vi "Position Arming LED.vi"(8 "error in (no error)":errorcluster, 9 "GPS Status LED":refnum<vi>, 10 "Aircraft Id Ref":refnum<vi>, 11 "LED Ref":refnum<vi>) -> (0 "error out":errorcluster)   [LabVIEW 2014]
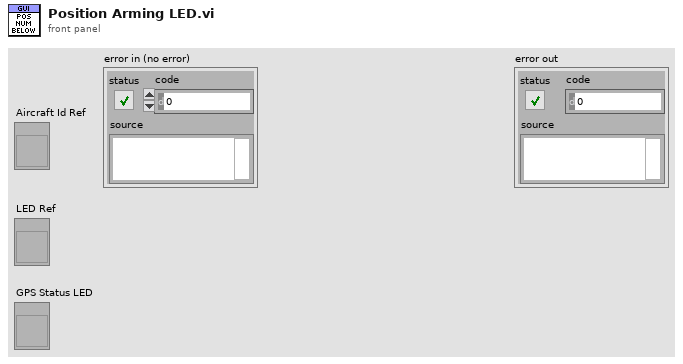
[diagram p1: front panel]
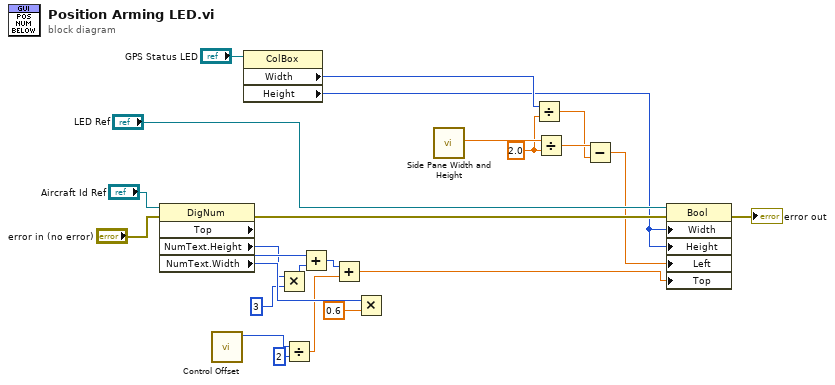
[diagram p0: block diagram]
diagram:
  w4 = 2.0 ("y")
  n1 = property class="DigNum"(reference="Aircraft Id Ref", error in="error in (no error)") -> (error out=w24:errorcluster, "Top"=w23:i32, "NumText.Height"=w14:u32, "NumText.Width"=w19:u32)  [unwired: 1 out]
  n2 = call "Control Offset.vi"() -> ("Offset From Tab Edge in (px)"=w10:i32)  [unwired: 11 in]
  n3 = property class="ColBox"(reference="GPS Status LED") -> ("Width"=w5:u32, "Height"=w1:u32)  [unwired: 1 in, 2 out]
  n4 = Multiply(x=w14, y=u32 3) -> (x*y=w13:u32)
  n5 = Divide(x=w10, y=2) -> (x/y=w8:dbl)
  n6 = Add(x=w23, y=w13) -> (x+y=w22:u32)
  n7 = Add(x=w22, y=w8) -> (x+y=w15:dbl)
  n8 = Multiply(x=w19, y=0.6) -> ()  [unwired: 1 out]
  n9 = call "Side Pane Width and Height.vi"() -> ("Width"=w7:dbl)  [unwired: 9 in, 2 out]
  n10 = Divide(x=w5, y=w4) -> (x/y=w3:dbl)
  n11 = Divide(x=w7, y=w4) -> (x/y=w6:dbl)
  n12 = Subtract(x=w6, y=w3) -> (x-y=w2:dbl)
  n13 = property class="Bool"(reference="LED Ref", error in=w24, "Width"=w1, "Height"=w1, "Left"=w2, "Top"=w15) -> (error out=→"error out":errorcluster)  [unwired: 1 out]
